vi "CANBootloader.vi"() -> ()   [LabVIEW 2010]
uses:
  <vilib>/Utility/miscctls.llb/LVRowAndColumnTypeDef.ctl
  USB2XXX.dll
panel:
  in  "pCRC16":u16
  in  "pBufferSize":u16
  in  "pFWType":u8
  in  "pFWVersion":u32
  in  "CAN Index":i32(ring) items=["0", "1"]
  in  "BaudRate":i32=1000000
  in  "IDType":u8
  in  "ReceiveDataID":u32=61 format="%x"
  in  "SendDataID":u32=60 format="%x"
  out "NodeAddr":i32
  out "pVersion out":u32
  out "Node Position":T1
  in  "Device Index":i32(ring) items=["0", "1", "2", "3", "4", "5"]
  out "固件更新进度":i32(slide) scale=0.0..4284.0
  in  "Upgrate":bool
  out "NodeNum":u16
  in  "扫描节点":bool
  out "扫描进度":u16(slide) max=9 scale=0.0..299.0
  in  "EndAddr":u16=255
  in  "StartAddr":u16=1
  in  "Table Scan Node":string[][](table)
  in  "stop":bool
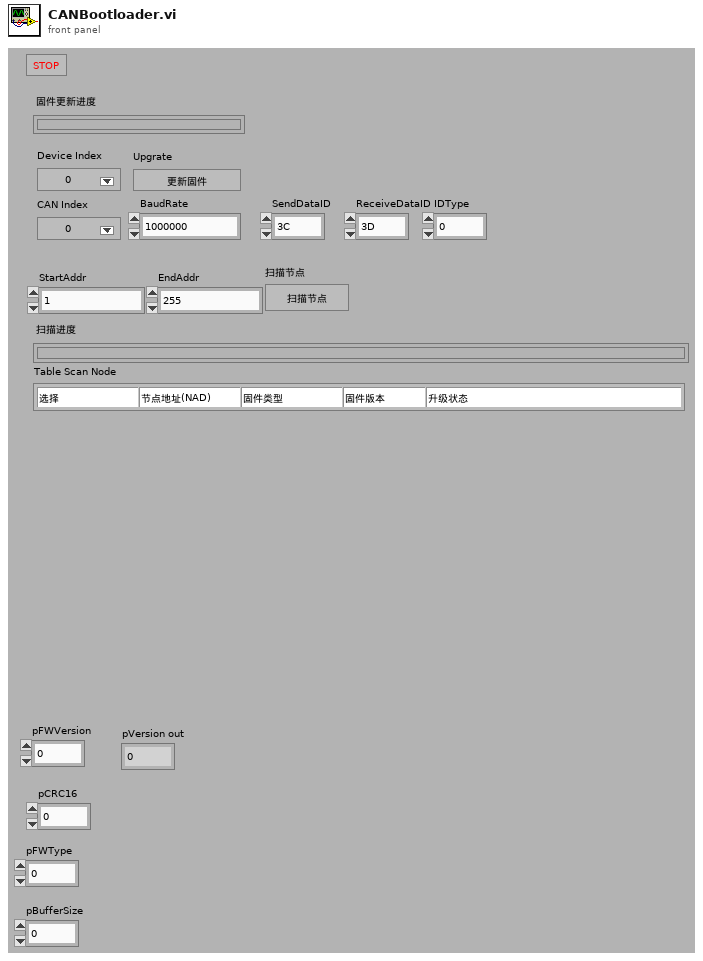
[diagram p1: front panel]
types:
  T1 = typedef "LVRowAndColumnTypeDef.ctl" = cluster{"Row":i32, "Column":i32}
  T2 = enum16{"Init", "ScanNode", "Upgrate", "Colse", "Idel"}
  T3 = typedef "LVPoint32TypeDef.ctl" = cluster{"Horizontal":i32, "Vertical":i32}
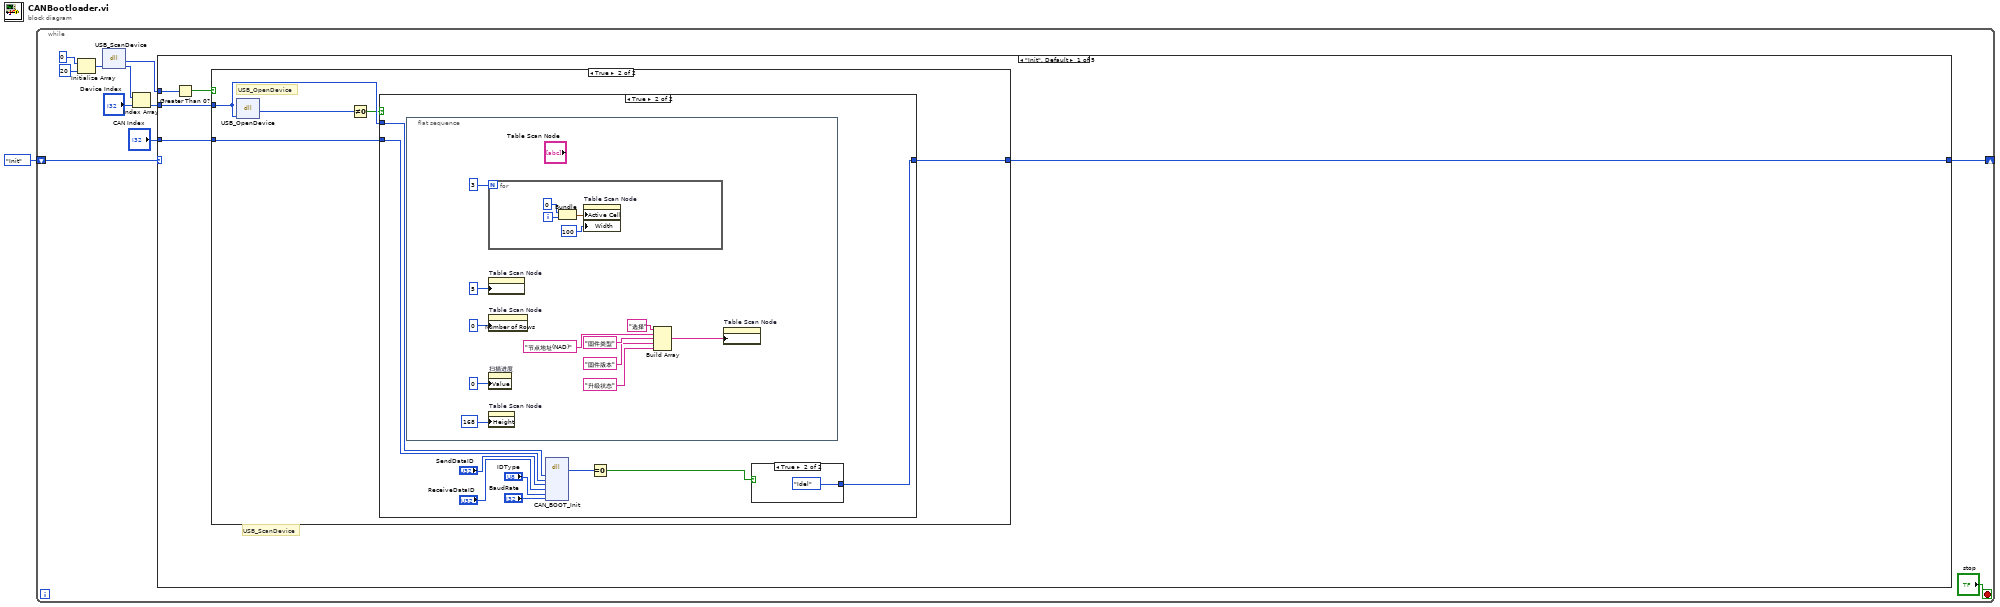
[diagram p0: block diagram]
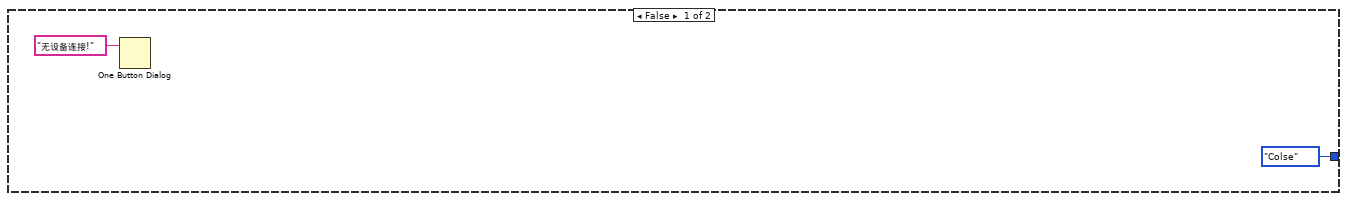
[diagram p2: hidden frame]
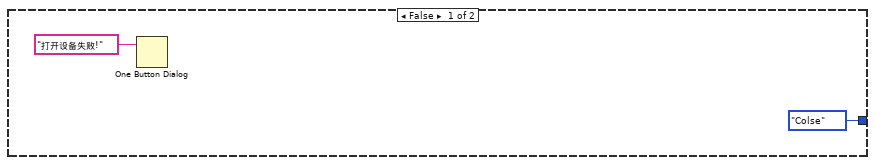
[diagram p3: hidden frame]
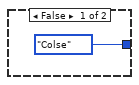
[diagram p4: hidden frame]
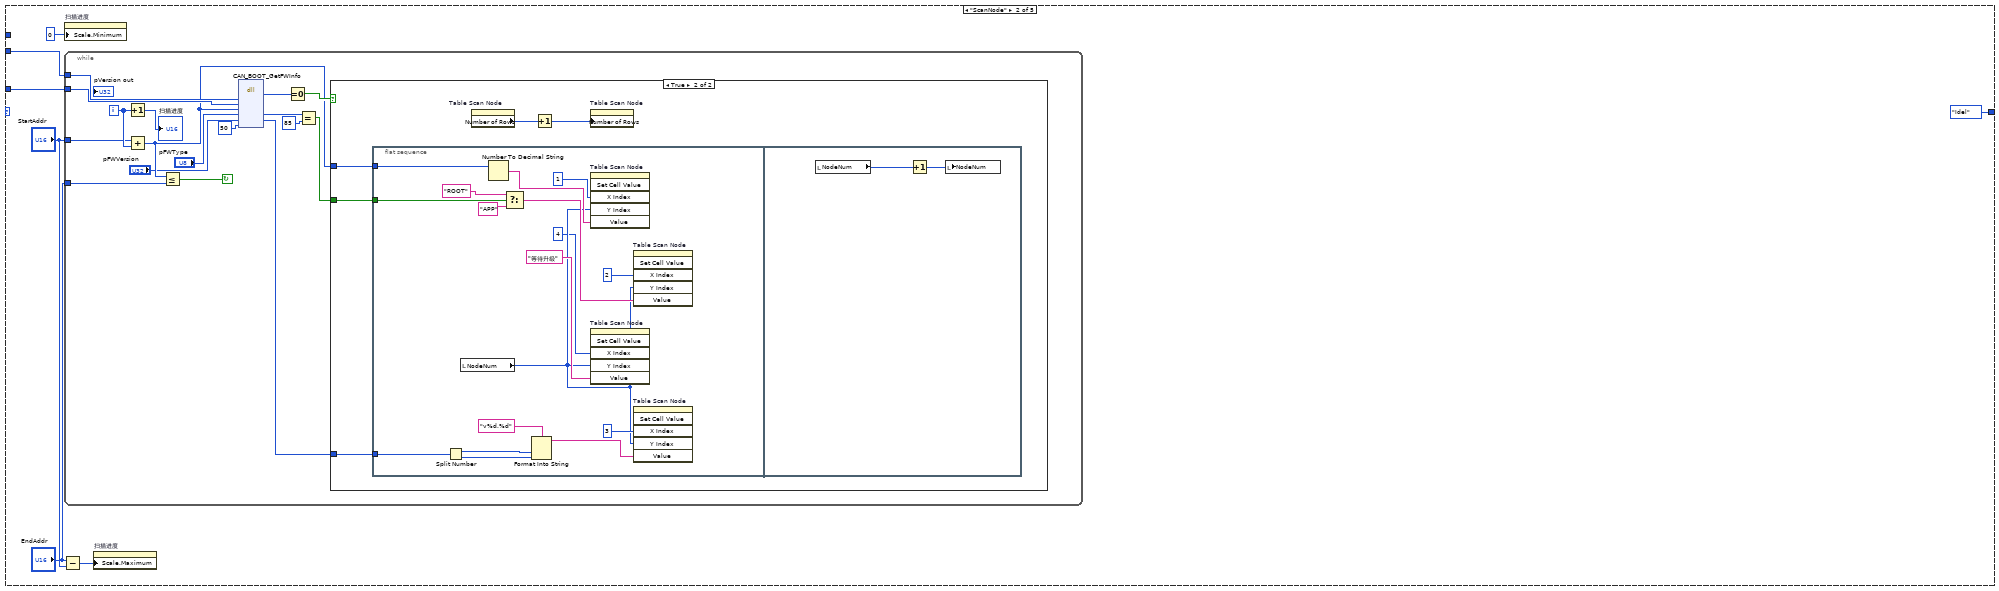
[diagram p5: hidden frame]
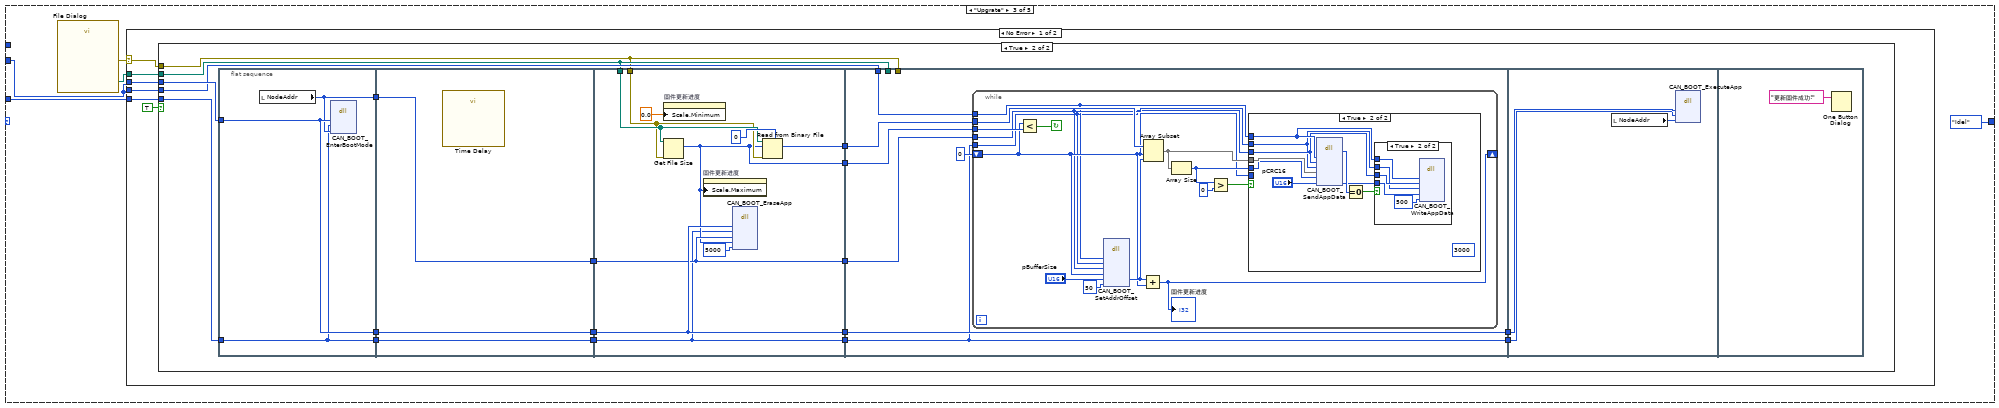
[diagram p7: hidden frame]
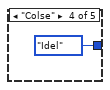
[diagram p12: hidden frame]
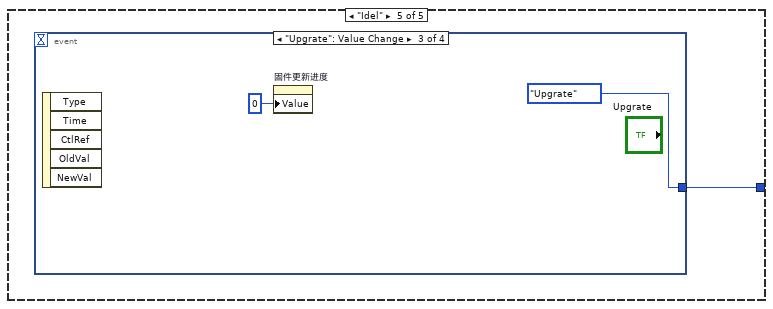
[diagram p13: hidden frame]
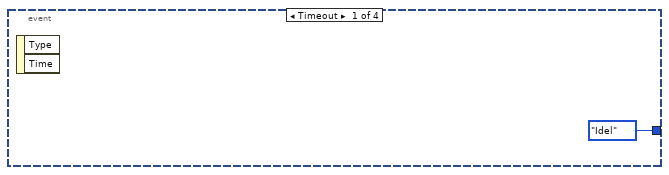
[diagram p14: hidden frame]
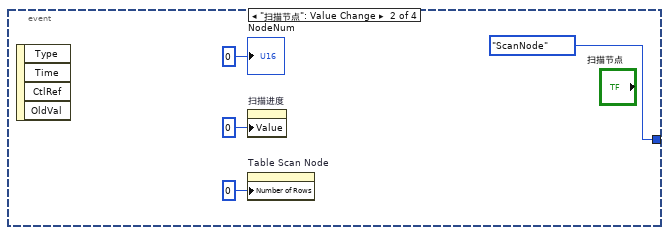
[diagram p15: hidden frame]
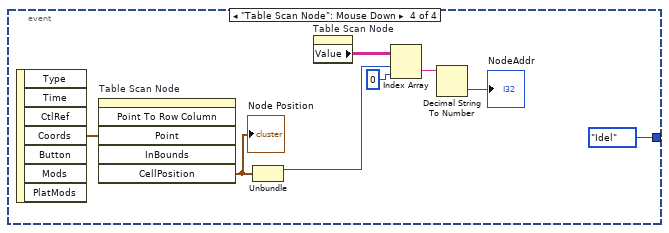
[diagram p16: hidden frame]
diagram:
  n1 = while {
    shift-right: [w10] -> _
    shift-left: T2."Init" ("Enum") -> [w11]
    stop <- "stop" stop-if-true
    n2 = Initialize Array(0, 20 ("dimension size")) -> (w7:i32[])
    n3 = dll-call lib="E:/OtherWork/STM32/USB2XXX_Example/trunk/Labview/USB2CAN/CANBootloader/USB2XXX.dll" fn="USB_ScanDevice"("pDevNum"=w7) -> ("return type"=w3:i32, "pDevNum"=w8:i32[])  [unwired: 3 in, 2 out]
    n4 = Index Array(array=w8, index="Device Index") -> (element=w4:i32)
    n5 = case shown="\"Init\", Default" w11 {
      tunnel: [w16 T2."Idel" ("Enum") T2."Idel" ("Enum") T2."Idel" ("Enum") w187] -> w10
      tunnel: w4 -> [w15 w56 w102 _ _]
      tunnel: w3 -> [w14 _ _ _ _]
      tunnel: "CAN Index" -> [w13 w53 w101 _ _]
      frame "Init", Default {
        # "USB_ScanDevice"
        n6 = Greater Than 0?(x=w14) -> (x > 0?=w17:bool)
        n7 = case shown="True" w17 {
          tunnel: [T2."Colse" ("Enum") w23] -> w16
          tunnel: w15 -> [_ w22]
          tunnel: w13 -> [_ w20]
          frame False {
            n8 = One Button Dialog(message="无设备连接!") -> ()  [unwired: 1 in, 1 out]
          }
          frame True {
            # "USB_OpenDevice"
            n9 = dll-call lib="E:/OtherWork/STM32/USB2XXX_Example/trunk/Labview/USB2CAN/CANBootloader/USB2XXX.dll" fn="USB_OpenDevice"("DevIndex"=w22) -> ("return type"=w24:u8)  [unwired: 4 in, 2 out]
            n10 = Not Equal To 0?(x=w24) -> (x != 0?=w21:bool)
            n11 = case shown="True" w21 {
              tunnel: [T2."Colse" ("Enum") w34] -> w23
              tunnel: w22 -> [_ w28]
              tunnel: w20 -> [_ w27]
              frame False {
                n12 = One Button Dialog(message="打开设备失败!") -> ()  [unwired: 1 in, 1 out]
              }
              frame True {
                n13 = flat-sequence {
                  frame #0 {
                    n14 = for {
                      N: 3 -> [_]
                      i -> [w52]
                      n15 = Bundle("Number of Rows"=u32 0, w52) -> (w50:cluster{"Number of Rows":u32, i32})  [unwired: 1 in]
                      n16 = property on="Table Scan Node" class="Tbl (strict)"("Active Cell"=w50, "Width"=u32 100 ("Active Cell:Cell Size:Width")) -> ()  [unwired: 2 in, 2 out]
                    }
                    n17 = property on="Table Scan Node" class="Tbl (strict)"("Number of Columns"=u32 5) -> ()  [unwired: 2 in, 2 out]
                    n18 = property on="Table Scan Node" class="Tbl (strict)"("Number of Rows"=u32 0) -> ()  [unwired: 2 in, 2 out]
                    n19 = property on="扫描进度" class="Slide (strict)"("Value"=u16 0 ("扫描进度")) -> ()  [unwired: 2 in, 2 out]
                    n20 = property on="Table Scan Node" class="Tbl (strict)"("Height"=u32 168 ("Size:Height")) -> ()  [unwired: 2 in, 2 out]
                    n21 = Build Array("选择", "节点地址(NAD)", "固件类型", "固件版本", "升级状态") -> (w46:string[])
                    n22 = property on="Table Scan Node" class="Tbl (strict)"("Column Headers[]"=w46) -> ()  [unwired: 2 in, 2 out]
                  }
                }
                n23 = dll-call lib="E:/OtherWork/STM32/USB2XXX_Example/trunk/Labview/USB2CAN/CANBootloader/USB2XXX.*" fn="CAN_BOOT_Init"("DevHandle"=w28, "CANIndex"=w27, "SendDataID"="SendDataID", "ReceiveDataID"="ReceiveDataID", "IDType"="IDType", "BaudRate"="BaudRate") -> (w29:i32)  [unwired: 9 in, 2 out]
                n24 = Equal To 0?(x=w29) -> (x = 0?=w35:bool)
                n25 = case shown="True" w35 {
                  tunnel: [T2."Colse" ("Enum") T2."Idel" ("Enum")] -> w34
                  frame False {
                  }
                  frame True {
                  }
                }
              }
            }
          }
        }
      }
      frame "ScanNode" {
        n26 = Subtract(x="EndAddr", y="StartAddr") -> (x-y=w58:u16)
        n27 = property on="扫描进度" class="Slide (strict)"("Scale.Minimum"=u8 0 ("Response to Value Outside Limits:Minimum")) -> ()  [unwired: 2 in, 2 out]
        n28 = while {
          tunnel: w56 -> [w68]
          tunnel: "StartAddr" -> [w72]
          tunnel: "EndAddr" -> [w71]
          tunnel: w53 -> [w66]
          i -> [w74]
          stop <- w73 continue-if-true
          n29 = Increment(x=w74) -> (x+1=→"扫描进度":i32)
          n30 = Add(x=w72, y=w74) -> (x+y=w65:i32)
          n31 = Less Or Equal?(x=w65, y=w71) -> (x <= y?=w73:bool)
          n32 = dll-call lib="E:/OtherWork/STM32/USB2XXX_Example/trunk/Labview/USB2CAN/CANBootloader/USB2XXX.dll" fn="CAN_BOOT_GetFWInfo"("DevHandle"=w68, "CANIndex"=w66, "NAD"=w65, "pFWType"="pFWType", "pFWVersion"="pFWVersion", "TimeOutOfMs"=u32 50 ("TimeOut")) -> ("return type"=w67:i32, "pFWType"=w61:u8, "pFWVersion"=w60:u32)  [unwired: 7 in, 2 out]
          n33 = Equal To 0?(x=w67) -> (x = 0?=w75:bool)
          n34 = Equal?(x=w61, y=u32 85) -> (x = y?=w69:bool)
          n35 = case shown="True" w75 {
            tunnel: w65 -> [_ w81]
            tunnel: w69 -> [_ w78]
            tunnel: w60 -> [_ w77]
            frame False {
            }
            frame True {
              n36 = flat-sequence {
                tunnel: w81 -> [w94]
                tunnel: w78 -> [w91]
                tunnel: w77 -> [w89]
                frame #0 {
                  n37 = Split Number(x=w89) -> (hi(x)=w87:u16, lo(x)=w86:u16)
                  n38 = local read "NodeNum"() -> (w83:u16)
                  n39 = Number To Decimal String(number=w94) -> (decimal integer string=w98:string)  [unwired: 1 in]
                  n40 = Select(t="ROOT" ("Value"), s=w91, f="APP" ("Value")) -> (s? t:f=w90:string)
                  n41 = Format Into String(format string="v%d.%d", w87, w86) -> (resulting string=w85:string)  [unwired: 2 in, 1 out]
                  n42 = invoke on="Table Scan Node" class="Tbl (strict)" method="Set Cell Value"("X Index"=u32 1, "Y Index"=w83, "Value"=w98) -> ()  [unwired: 3 in, 6 out]
                  n43 = invoke on="Table Scan Node" class="Tbl (strict)" method="Set Cell Value"("X Index"=u32 4, "Y Index"=w83, "Value"="等待升级") -> ()  [unwired: 3 in, 6 out]
                  n44 = invoke on="Table Scan Node" class="Tbl (strict)" method="Set Cell Value"("X Index"=u32 2, "Y Index"=w83, "Value"=w90) -> ()  [unwired: 3 in, 6 out]
                  n45 = invoke on="Table Scan Node" class="Tbl (strict)" method="Set Cell Value"("X Index"=u32 3, "Y Index"=w83, "Value"=w85) -> ()  [unwired: 3 in, 6 out]
                }
                frame #1 {
                  n46 = local read "NodeNum"() -> (w100:u16)
                  n47 = Increment(x=w100) -> (x+1=w99:u16)
                  n48 = local write "NodeNum"(w99) -> ()
                }
              }
              n49 = property on="Table Scan Node" class="Tbl (strict)"() -> ("Number of Rows"=w79:u32)  [unwired: 2 in, 2 out]
              n50 = Increment(x=w79) -> (x+1=w80:u32)
              n51 = property on="Table Scan Node" class="Tbl (strict)"("Number of Rows"=w80) -> ()  [unwired: 2 in, 2 out]
            }
          }
        }
        n52 = property on="扫描进度" class="Slide (strict)"("Scale.Maximum"=w58) -> ()  [unwired: 2 in, 2 out]
      }
      frame "Upgrate" {
        n53 = call "File Dialog"() -> ("selected path"=w103:path, "error out"=w104:errorcluster)  [unwired: 12 in, 2 out]
        n54 = case shown="No Error" w104 {
          selector: w104 -> [w108 _]
          tunnel: w103 -> [w109 _]
          tunnel: w102 -> [w111 _]
          tunnel: w102 -> [w110 _]
          tunnel: w101 -> [w107 _]
          frame No Error {
            n55 = case shown="True" TRUE {
              tunnel: w111 -> [_ w117]
              tunnel: w110 -> [_ w116]
              tunnel: w109 -> [_ w115]
              tunnel: w108 -> [_ w114]
              tunnel: w107 -> [_ w113]
              frame False {
              }
              frame True {
                n56 = flat-sequence {
                  tunnel: w117 -> [w132]
                  tunnel: [w131] -> w129
                  tunnel: [w132] -> w128
                  tunnel: w113 -> [w130]
                  tunnel: [w130] -> w127
                  tunnel: w129 -> [w135]
                  tunnel: [w135] -> w126
                  tunnel: w128 -> [w134]
                  tunnel: [w134] -> w125
                  tunnel: w127 -> [w133]
                  tunnel: [w133] -> w124
                  tunnel: w126 -> [w139]
                  tunnel: [w139] -> w123
                  tunnel: w125 -> [w140]
                  tunnel: w115 -> [w144]
                  tunnel: w114 -> [w143]
                  tunnel: [w142] -> w122
                  tunnel: [w138] -> w121
                  tunnel: [w140] -> w120
                  tunnel: w124 -> [w136]
                  tunnel: [w136] -> w119
                  tunnel: w115 -> [_]
                  tunnel: w114 -> [_]
                  tunnel: w116 -> [w151]
                  tunnel: w123 -> [w150]
                  tunnel: w122 -> [w149]
                  tunnel: w121 -> [w148]
                  tunnel: [w147] -> w118
                  tunnel: w120 -> [w147]
                  tunnel: w119 -> [w146]
                  tunnel: [w146] -> w112
                  tunnel: w118 -> [w184]
                  tunnel: w112 -> [w182]
                  frame #0 {
                    n57 = local read "NodeAddr"() -> (w131:i32)
                    n58 = dll-call lib="E:/OtherWork/STM32/USB2XXX_Example/trunk/Labview/USB2CAN/CANBootloader/USB2XXX.*" fn="CAN_BOOT_EnterBootMode"("DevHandle"=w132, "CANIndex"=w130, "NAD"=w131) -> ()  [unwired: 7 in, 2 out]
                  }
                  frame #1 {
                    n59 = call "Time Delay"() -> ()  [unwired: 11 in, 1 out]
                  }
                  frame #2 {
                    n60 = property on="固件更新进度" class="Slide (strict)"("Scale.Minimum"=0.0 ("Scale.Range:Minimum")) -> ()  [unwired: 2 in, 2 out]
                    n61 = Get File Size(file=w144, error in=w143) -> (size (in bytes)=w138:i64)  [unwired: 2 out]
                    n62 = property on="固件更新进度" class="Slide (strict)"("Scale.Maximum"=w138) -> ()  [unwired: 2 in, 2 out]
                    n63 = dll-call lib="E:/OtherWork/STM32/USB2XXX_Example/trunk/Labview/USB2CAN/CANBootloader/USB2XXX.*" fn="CAN_BOOT_EraseApp"("DevHandle"=w140, "CANIndex"=w136, "NAD"=w139, "AppSizeOfByte"=w138, "TimeOutOfMs"=u32 5000 ("TimeOut")) -> ()  [unwired: 9 in, 2 out]
                    n64 = Read from Binary File(5:u8 0, 8:w143, 10:w138, 11:w144) -> (2:w142:u8[])  [unwired: 2 in, 3 out]
                  }
                  frame #3 {
                    n65 = while {
                      shift-right: [w160] -> _
                      shift-left: 0 -> [w156]
                      tunnel: w148 -> [w166]
                      tunnel: w149 -> [w165]
                      tunnel: w151 -> [w154]
                      tunnel: w150 -> [w155]
                      tunnel: w146 -> [w153]
                      stop <- w167 continue-if-true
                      n66 = Less?(x=w156, y=w166) -> (x < y?=w167:bool)
                      n67 = dll-call lib="E:/OtherWork/STM32/USB2XXX_Example/trunk/Labview/USB2CAN/CANBootloader/USB2XXX.*" fn="CAN_BOOT_SetAddrOffset"("DevHandle"=w154, "CANIndex"=w153, "NAD"=w155, "AddrOffset"=w156, "pBufferSize"="pBufferSize", "TimeOutOfMs"=u32 50) -> ("pBufferSize"=w159:u16)  [unwired: 9 in, 2 out]
                      n68 = Add(x=w159, y=w156) -> (x+y=w160:i32)
                      "固件更新进度" <- w160
                      n69 = Array Subset(array=w165, index=w156, length=w159) -> (w161:u8[])
                      n70 = Array Size(array=w161) -> (size(s)=w162:i32)
                      n71 = Greater?(x=w162, y=0) -> (0:w163:bool)
                      n72 = case shown="True" w163 {
                        tunnel: w162 -> [_ w174]
                        tunnel: w154 -> [_ w170]
                        tunnel: w155 -> [_ w168]
                        tunnel: w156 -> [_ _]
                        tunnel: w161 -> [_ w175]
                        tunnel: w153 -> [_ w169]
                        frame False {
                        }
                        frame True {
                          (unwired) u32 3000 ("TimeOut")
                          n73 = dll-call lib="E:/OtherWork/STM32/USB2XXX_Example/trunk/Labview/USB2CAN/CANBootloader/USB2XXX.*" fn="CAN_BOOT_SendAppData"("DevHandle"=w170, "CANIndex"=w169, "NAD"=w168, "pData"=w175, "DataLen"=w174, "pCRC16"="pCRC16") -> (w173:i32, "pCRC16"=w171:u16)  [unwired: 8 in, 2 out]
                          n74 = Equal To 0?(x=w173) -> (x = 0?=w172:bool)
                          n75 = case shown="True" w172 {
                            tunnel: w171 -> [_ w181]
                            tunnel: w170 -> [_ w179]
                            tunnel: w169 -> [_ w178]
                            tunnel: w168 -> [_ w177]
                            frame False {
                            }
                            frame True {
                              n76 = dll-call lib="E:/OtherWork/STM32/USB2XXX_Example/trunk/Labview/USB2CAN/CANBootloader/USB2XXX.*" fn="CAN_BOOT_WriteAppData"("DevHandle"=w179, "CANIndex"=w178, "NAD"=w177, "CRC16"=w181, "TimeOutOfMs"=u32 500) -> ()  [unwired: 9 in, 2 out]
                            }
                          }
                        }
                      }
                    }
                  }
                  frame #4 {
                    n77 = local read "NodeAddr"() -> (w183:i32)
                    n78 = dll-call lib="E:/OtherWork/STM32/USB2XXX_Example/trunk/Labview/USB2CAN/CANBootloader/USB2XXX.*" fn="CAN_BOOT_ExecuteApp"("DevHandle"=w184, "CANIndex"=w182, "NAD"=w183) -> ()  [unwired: 7 in, 2 out]
                  }
                  frame #5 {
                    n79 = One Button Dialog(message="更新固件成功!") -> ()  [unwired: 1 in, 1 out]
                  }
                }
              }
            }
          }
          frame Error {
          }
        }
      }
      frame "Colse" {
      }
      frame "Idel" {
        n80 = event shown="[2] \"Upgrate\": Value Change" {
          selector: _ -> [_ _ _ _]
          dyn-events: _ -> [_ _ _ _]
          timeout: _ -> [_ _ _ _]
          tunnel: [T2."Idel" ("Enum") T2."ScanNode" ("Enum") T2."Upgrate" ("Enum") T2."Idel" ("Enum")] -> w187
          event Timeout {
            n81 = event-data() -> ()  [unwired: 1 in, 2 out]
          }
          event "扫描节点": Value Change {
            n82 = event-data() -> ()  [unwired: 1 in, 4 out]
            n83 = property on="扫描进度" class="Slide (strict)"("Value"=u16 0 ("扫描进度")) -> ()  [unwired: 2 in, 2 out]
            n84 = property on="Table Scan Node" class="Tbl (strict)"("Number of Rows"=u32 0) -> ()  [unwired: 2 in, 2 out]
            "NodeNum" <- u16 0 ("NodeNum")
          }
          event "Upgrate": Value Change {
            n85 = event-data() -> ()  [unwired: 1 in, 5 out]
            n86 = property on="固件更新进度" class="Slide (strict)"("Value"=u8 0 ("固件更新进度")) -> ()  [unwired: 2 in, 2 out]
          }
          event "Table Scan Node": Mouse Down {
            n87 = event-data() -> ("Coords"=w202:T3)  [unwired: 1 in, 6 out]
            n88 = invoke on="Table Scan Node" class="Tbl (strict)" method="Point To Row Column"("Point"=w202) -> ("CellPosition"=w199:T1)  [unwired: 5 in, 5 out]
            "Node Position" <- w199
            n89 = Unbundle(w199) -> ("Row"=w198:i32)  [unwired: 1 out]
            n90 = property on="Table Scan Node" class="Tbl (strict)"() -> ("Value"=w200:string[][])  [unwired: 2 in, 2 out]
            n91 = Index Array(array=w200, index (row)=w198, index (col)=0 ("disabled index (col)")) -> (element=w196:string)
            n92 = Decimal String To Number(string=w196) -> (number=→"NodeAddr":i32)  [unwired: 2 in, 1 out]
          }
        }
      }
    }
  }
